vi "ReadMovieFrame.vi"(3 "error in":errorcluster, 4 "Frame Number":i32, 5 "QT Ref In":T1) -> (0 "error out":errorcluster, 1 "Image Out":T2 {"Dialogs" format="%.0b"}, 2 "QT Ref Out":T1)   [LabVIEW 2024]
doc: "This VI works with the OpenMovieFile.vi. Once the QT Ref Out wire is connected from the OpenMovieFile.vi and a frame number is specified, this vi will return the appropriate image from the movie file."
uses:
  <userlib>/ImageProcessing/QTLIB_2595_LV86/QT_Private.ctl
  <userlib>/ImageProcessing/QTLIB_2595_LV86/QT_FrameSelector.ctl
  <userlib>/ImageProcessing/QTLIB_2595_LV86/QT_Image.ctl
  <userlib>/ImageProcessing/QTLIB_2595_LV86/QT_Ref.ctl
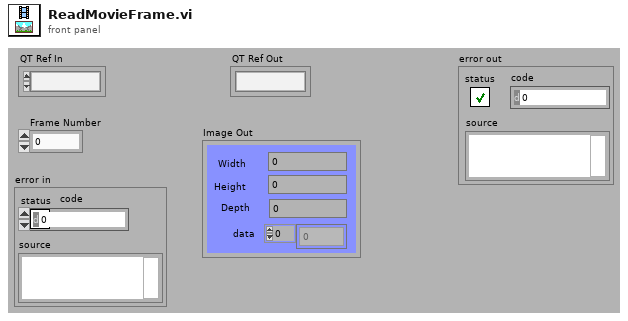
[diagram p1: front panel]
types:
  T1 = typedef "QT_Ref.ctl" = refnum<k1>
  T2 = typedef "QT_Image.ctl" = cluster{"Width":i32, "Height":i32, "Depth":i32, "data":u8[], "Compressed data":u8[], "Color table":u32[], "Duration":i32, "Options":i32, "Timestamp":i32, "ID":i32, "Reserved":i32, "Dialogs":u32}
  T3 = typedef "QT_FrameSelector.ctl" = enum32{"Get Next Frame", "Get Prev Frame", "Get Last Frame", "Get First Frame", "Get Frame ID", "Get Frame at Time", "reserved"}
  T4 = typedef "QT_Private.ctl" = cluster{"reserved 1":i32, "reserved 2":i32, "reserved 3":i32, "reserved 4":i32}
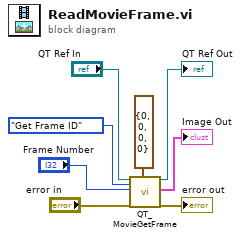
[diagram p0: block diagram]
diagram:
  n1 = call <userlib>:"QT_MovieGetFrame.vi"("QT Ref In"="QT Ref In", "Frame Access"=QT_FrameSelector."Get Frame ID", "Frame ID"="Frame Number", "error in"="error in", "Private"=T4 {"reserved 1"=0, "reserved 2"=0, "reserved 3"=0, "reserved 4"=0}) -> ("QT Ref Out"=→"QT Ref Out":T1, "Image Out"=→"Image Out":T2, "error out"=→"error out":errorcluster)  [unwired: 12 out]
